vi "Read Multi I16.vi"(8 "error in (no error)":errorcluster, 9 "Type":i16[](array[numeric]), 10 "Tag":string[](array[string]), 11 "Var Bus in":refnum<class "Omni_Bus.lvclass">) -> (0 "error out":errorcluster, 2 "I16's":i16[](array[numeric]), 3 "Var Bus out":refnum<class "Omni_Bus.lvclass">)   [LabVIEW 2021, in "Omni_Bus.lvclass"]
uses:
  Omni_Bus.lvclass
  <vilib>/TSA/Abstract Data Classes/Abs_Types/I16 Integer/Abs_I16 Integer.lvclass
  C:/Program Files (x86)/National Instruments/LabVIEW 2021/vi.lib/TSA/Abstract Data Classes/Abs_Types/Type/Abs_Type.lvclass
  <vilib>/TSA/Abstract Data Classes/Abs_Types/Type/Abs_Type.lvclass/Abs_Type.ctl
  Omni_Bus.lvclass/Omni_Bus.ctl
  FindMultiVar.vi
  FindVar.vi
  <vilib>/Utility/error.llb/Clear Errors.vi
  Properties/Read Var Map.vi
  <vilib>/TSA/Abstract Data Classes/Abs_Types/Type/Properties/Read Tag.vi
  <vilib>/TSA/Abstract Data Classes/Abs_Types/Value/Abs_Value.lvclass
  Check For Read Only Error.vi
  Incorrect Tag String Error.vi
  <vilib>/TSA/Abstract Data Classes/Abs_Types/Type/Abs_Type.lvclass
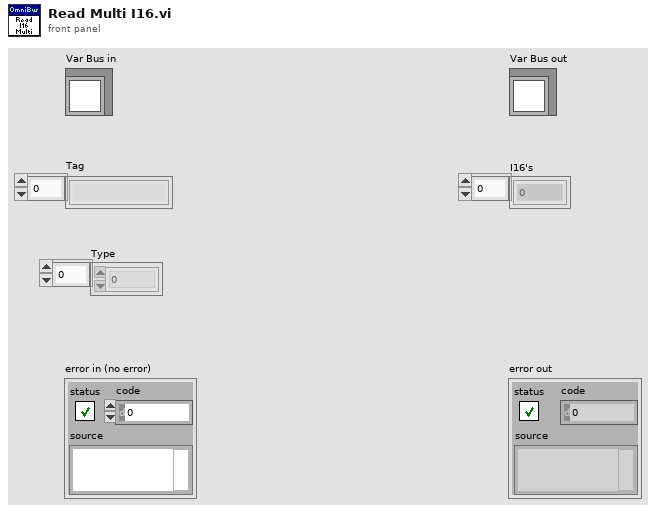
[diagram p1: front panel]
types:
  T1 = typedef "Abs_I16 Integer.lvclass/Type.ctl" = i16
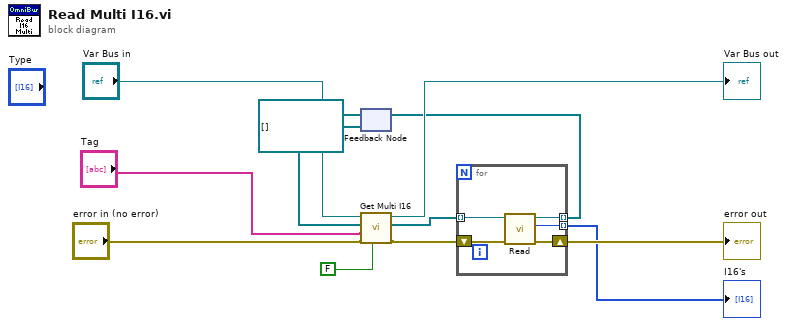
[diagram p0: block diagram]
diagram:
  n1 = feedback #1(refnum<class "Abs_I16 Integer.lvclass">[] []) -> (w3:refnum<class "Abs_I16 Integer.lvclass">[])
  n2 = call "Get Multi I16.vi"("Write?"=FALSE, "error in (no error)"="error in (no error)", "Tag"="Tag", "Value Type"=w3, "Var Bus in"="Var Bus in") -> ("error out"=w5:errorcluster, "Value Out"=w4:refnum<class "Abs_I16 Integer.lvclass">[], "Var Bus out"=→"Var Bus out":refnum<class "Omni_Bus.lvclass">)  [unwired: 3 in, 1 out]
  n3 = for {
    tunnel: [w16] -> w7 mode=indexing
    tunnel: [w15] -> w6 mode=indexing
    tunnel: w4 -> [w13] mode=indexing
    shift-right: [w17] -> w11
    shift-left: w5 -> [w14]
    n4 = call-dynamic "Read.vi"("error in (no error)"=w14, "Double Float.lvclass_340760 in"=w13) -> ("error out"=w17:errorcluster, "Value"=w16:T1, "Double Float.lvclass_340760 out"=w15:refnum<class "Abs_I16 Integer.lvclass">)  [unwired: 7 in]
  }
  "error out" <- w11
  "I16's" <- w7
  n5 = feedback-in #1(w6) -> ()
